vi "Read Holding Register.vi"(8 "error in (no error)":errorcluster, 9 "number of inputs":u16, 10 "starting address":u16, 11 "Modbus in":refnum<class "Modbus.lvclass">) -> (0 "error out":errorcluster, 2 "register values":u16[](array[numeric]), 3 "Modbus out":refnum<class "Modbus.lvclass">)   [LabVIEW 2023, in "HardwareAbstractionLayer_LVOOP.lvlib" / "Modbus.lvclass"]
uses:
  Modbus.lvclass
  Modbus.lvclass/Modbus.ctl
  <vilib>/NI/Modbus Library/API/Master/Modbus Master.lvclass
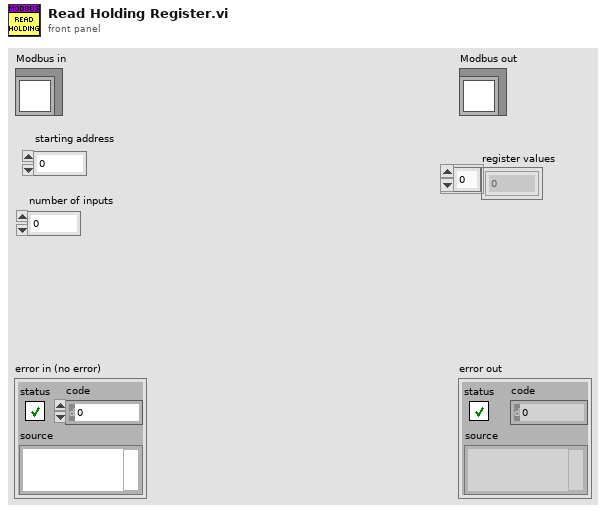
[diagram p1: front panel]
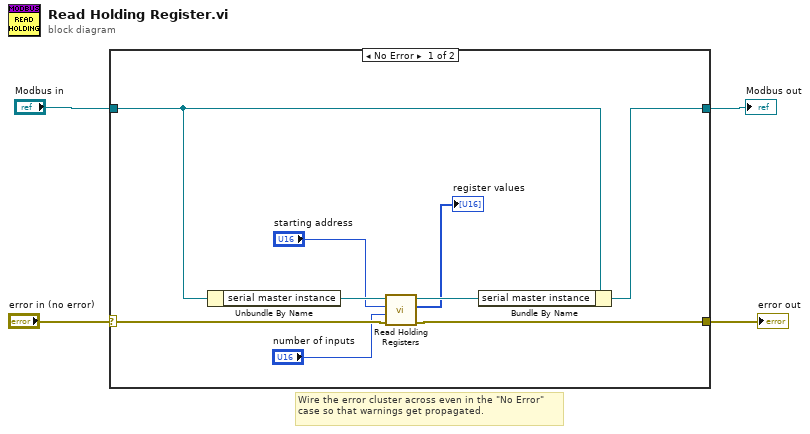
[diagram p0: block diagram]
diagram:
  # "Wire the error cluster across even in the \"No Error\"\ncase so that warnings get propagated."
  n1 = case shown="No Error" "error in (no error)" {
    selector: "error in (no error)" -> [w13 w15]
    tunnel: [w12 w15] -> w3
    tunnel: [w9 w14] -> w1
    tunnel: "Modbus in" -> [w10 w14]
    frame No Error {
      n2 = Unbundle By Name(w10) -> ("serial master instance"=w11:refnum<class "Modbus Master.lvclass">)
      n3 = call-dynamic "Read Holding Registers.vi"("error in"=w13, "number of inputs"="number of inputs", "starting address"="starting address", "Modbus master in"=w11) -> ("error out"=w12:errorcluster, "register values"=→"register values":u16[], "Modbus master out"=w8:refnum<class "Modbus Master.lvclass">)  [unwired: 5 in]
      n4 = Bundle By Name(cluster=w10, "serial master instance"=w8) -> (w9:refnum<class "Modbus.lvclass">)
    }
    frame Error {
    }
  }
  "error out" <- w3
  "Modbus out" <- w1
